vi "RobotMotionCommands2Dashboard.vi"(10 "Label":string="data", 11 "Robot Motion Commands":T1) -> ()   [LabVIEW 2018]
uses:
  Robot Pivot Motion Commands.ctl
  Pivot Motor Commands.ctl
  Robot Drive Mode.ctl
  <vilib>/Rock Robotics/Network Tables/NT Write Number.vi
  <vilib>/Rock Robotics/Network Tables/NT Write String.vi
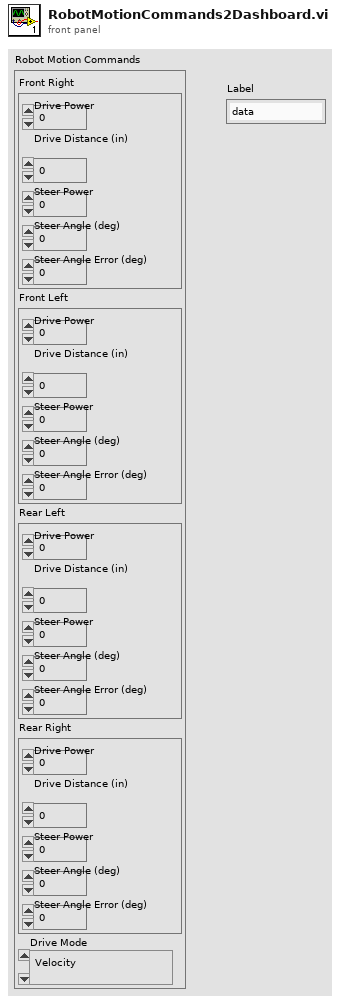
[diagram p1: front panel]
types:
  T1 = typedef "Robot Pivot Motion Commands.ctl" = cluster{"Front Right":T2, "Front Left":T2, "Rear Left":T2, "Rear Right":T2, "Drive Mode":T3}
  T2 = typedef "Pivot Motor Commands.ctl" = cluster{"Drive Power":dbl, "Drive Distance (in)":dbl, "Steer Power":dbl, "Steer Angle (deg)":dbl, "Steer Angle Error (deg)":dbl}
  T3 = typedef "Robot Drive Mode.ctl" = enum16{"Velocity", "Distance"}
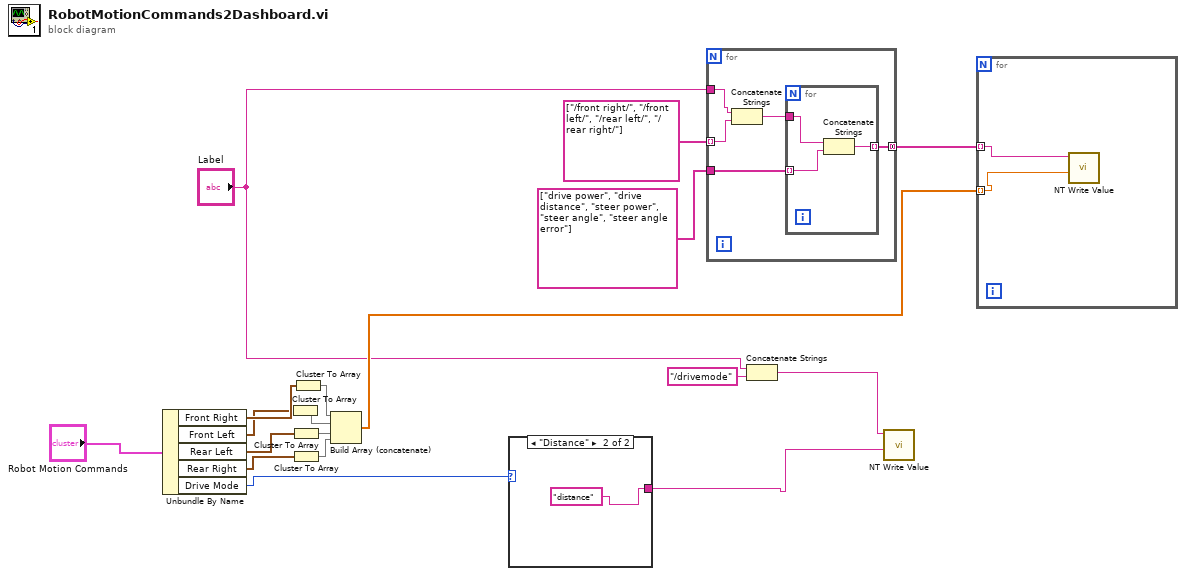
[diagram p0: block diagram]
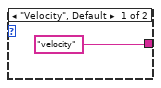
[diagram p2: hidden frame]
diagram:
  n1 = Unbundle By Name("Robot Motion Commands") -> ("Front Right"=w13:T2, "Front Left"=w9:T2, "Rear Left"=w8:T2, "Rear Right"=w11:T2, "Drive Mode"=w5:T3)
  n2 = Cluster To Array(cluster=w9) -> (array=w7:dbl[])
  n3 = Cluster To Array(cluster=w8) -> (array=w6:dbl[])
  n4 = Cluster To Array(cluster=w11) -> (array=w10:dbl[])
  n5 = Cluster To Array(cluster=w13) -> (array=w12:dbl[])
  n6 = Build Array (concatenate)(w12, w7, w6, w10) -> (w14:dbl[])
  n7 = case shown="\"Distance\"" w5 {
    tunnel: ["velocity" ("Label") "distance" ("Label")] -> w4
    frame "Velocity", Default {
    }
    frame "Distance" {
    }
  }
  n8 = for {
    tunnel: "Label" -> [w25]
    tunnel: string[] ["/front right/", "/front left/", "/rear left/", "/rear right/"] ("Label") -> [w24] mode=indexing
    tunnel: string[] ["drive power", "drive distance", "steer power", "steer angle", "steer angle error"] ("Label") -> [w22]
    tunnel: [w21] -> w15 mode=concatenating
    n9 = Concatenate Strings(w25, w24) -> (w23:string)
    n10 = for {
      tunnel: w23 -> [w28]
      tunnel: w22 -> [w27] mode=indexing
      tunnel: [w26] -> w21 mode=indexing
      n11 = Concatenate Strings(w28, w27) -> (w26:string)
    }
  }
  n12 = Concatenate Strings("Label", "/drivemode" ("string")) -> (w1:string)
  n13 = call-poly <vilib>:"NT Write Value.vi"("String"=w4, "Name"=w1) -> ()  [unwired: 9 in, 1 out]
  n14 = for {
    tunnel: w15 -> [w30] mode=indexing
    tunnel: w14 -> [w29] mode=indexing
    n15 = call-poly <vilib>:"NT Write Value.vi"("Numeric"=w29, "Name"=w30) -> ()  [unwired: 9 in, 1 out]
  }
